vi "Test Set to Array.vi"() -> ()   [LabVIEW 2020]
uses:
  944aec28-58bb-4328-96b7-70fcfdaad198.vi
  000dc520-47cb-4f14-9cda-e2f88ec4e030.vi
  944aec28-58bb-4328-96b7-70fcfdaad198.vi/7c7783df-fd5a-49d9-9b7a-63cc9fb0e4e5.vi
  <vilib>/addons/_JKI Toolkits/Caraya/Caraya.lvlibp/1abvi3w/vi.lib/addons/_JKI Toolkits/Caraya/classes/Assert/Assert Equal Value and Type_Variant.vi
  <vilib>/addons/_JKI Toolkits/Caraya/Caraya.lvlibp/1abvi3w/vi.lib/addons/_JKI Toolkits/Caraya/classes/Test/Test.lvclass
  <vilib>/addons/_JKI Toolkits/Caraya/Caraya.lvlibp/1abvi3w/vi.lib/addons/_JKI Toolkits/Caraya/classes/Assert/Assert.lvclass
panel:
  out "error out":errorcluster
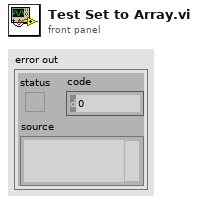
[diagram p1: front panel]
types:
  T1 = cluster{"Name":i32, "bool":bool, "string":string}[]
  T2 = set{cluster{"Name":i32, "bool":bool, "string":string}}
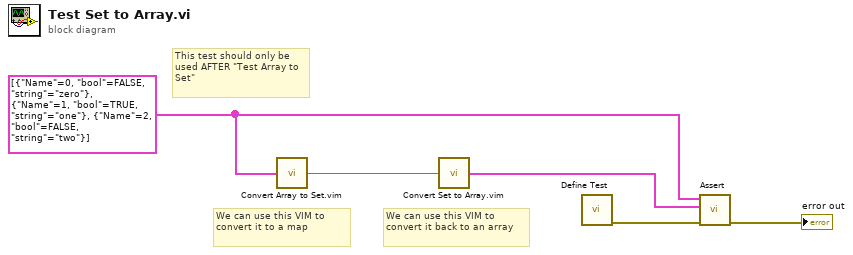
[diagram p0: block diagram]
diagram:
  w3 = T1 [{"Name"=0, "bool"=FALSE, "string"="zero"}, {"Name"=1, "bool"=TRUE, "string"="one"}, {"Name"=2, "bool"=FALSE, "string"="two"}] ("Array")
  # "We can use this VIM to convert it back to an array"
  # "This test should only be used AFTER \"Test Array to Set\""
  # "We can use this VIM to convert it to a map"
  n1 = call "Convert Array to Set.vim"("array"=w3) -> ("set"=w2:T2)  [unwired: 6 in]
  n2 = call "Convert Set to Array.vim"("set"=w2) -> ("array"=w1:T1)  [unwired: 8 in]
  n3 = call <vilib>:"Define Test.vi"() -> ("error out"=w4:errorcluster)  [unwired: 11 in]
  n4 = call-poly <vilib>:"Assert.vi"("error in (no error)"=w4, "Y"=w1, "X"=w3) -> ("error out"=→"error out":errorcluster)  [unwired: 8 in]
